vi "AutoExtracOpt.vi"() -> ()   [LabVIEW 2020]
uses:
  <vilib>/NI/Modbus Library/API/Master/Modbus Master.lvclass
  <vilib>/userdefined/High Color/IMAQdx.ctl
  subvi/status/StopSoftware.vi
  subvi/status/Tip_No_1000.vi
  subvi/status/Vial_No.vi
  subvi/status/Tip_No_300.vi
  subvi/status/Liquid_List.vi
  subvi/status/Log.vi
  subvi/status/LogCSVName.vi
  subvi/status/ExtracOptOperations.vi
  subvi/status/ExtracOptDeviceStatus.vi
  subvi/status/ExtracOptTaskStatus.vi
  subvi/status/ExtracOptTaskId.vi
  subvi/status/ExtracOptConversationId.vi
  subvi/status/EmergencyStop.vi
  subvi/status/ExtracOptCommand.vi
  subvi/HitBot/Robot-HL/small_scara_interface/small_scara_interface.lvlib
panel:
  out "ExtracOptDeviceStatus":string
  out "ExtracOptOperations":string
  out "ExtracOptConversationId":string
  out "ExtracOptTaskId":string
  out "Current_1000 uL_Tip_No":i32
  out "Current_300 uL_Tip_No":i32
  out "Current_Vial_No":i32
  out "Current_Log":string
  in  "Device_Log":i32(listbox)
  in  "StopSoftware":bool
  out "DK-CoverSwitcher_TCP":refnum<k5>
  out "DK-Gripper_TCP":refnum<class "Modbus Master.lvclass">
  in  "Control":enum32{"Auto", "Manual", "System", "Photo"}(tab)
  in  "9. End_Extraction 2":bool
  in  "9. End_Extraction":bool
  in  "8. Photo":bool
  in  "7. Shaker":bool
  in  "6. CoverSwitch_To_Extraction_Shaker":bool
  in  "5. CloseCover":bool
  in  "4. CoverSwitch_To_Vial_Storage":bool
  in  "3. OpenCover":bool
  in  "2. Vial_Storage_To_CoverSwitch":bool
  in  "1. DK-CoverSwitcher_Initial":bool
  in  "ExtracOptCommand 2":string="{\"organic_extractants\": [[\"A1\", 1.0], [\"A2\", 2.0]], \"aqueous_extractant\": [\"A3\", 1.0], \"additive\": [\"A4\", 0.0]}"
  in  "Tab Control":enum32{"HitBot76", "DK"}(tab)
  in  "HitBot76_ReadStatus":bool
  in  "HitBot76_Control":bool
  in  "HitBot76_Para":T1
  out "HitBot76_Status":T2
  in  "DK-Gripper_Control":bool
  in  "DK-Gripper_Para":cluster{"mode":string, "distance":i16}
  in  "DK-CoverSwitcher_Control":bool
  in  "DK-CoverSwitcher_Para":cluster{"mode":string}
  in  "PhotoCam":T3="cam1"
  in  "Change_Vial&Tip_No":bool
  in  "Vial_No":i32
  in  "Tip_No_1000":i32
  in  "Tip_No_300":i32
  out "Array":string[][](array[string])
  out "ExtracOptCommand":string
  in  "EmergencyStop":bool
  # "1-10"
  # "开盖模块初始化"
  # "将瓶子抓取到开盖模块，注意瓶子的当前编号"
  # "开瓶盖"
  # "将瓶子从开盖模块抓取回原处，注意瓶子的当前编号"
  # "关瓶盖"
  # "将瓶子从开盖模块抓取到萃取振荡平台"
  # "振荡"
  # "拍照"
  # "结束萃取"
  # "结束萃取"
  # "→ Y"
  # "mode = 0 正常运行\nmode = 1 切换坐标系\nmode = 2 控制夹爪 x\n表示行程0-20"
  # "89"
  # "1"
  # "4"
  # "2"
  # "→"
  # "→"
  # "1"
  # "3"
  # "8"
  # "96"
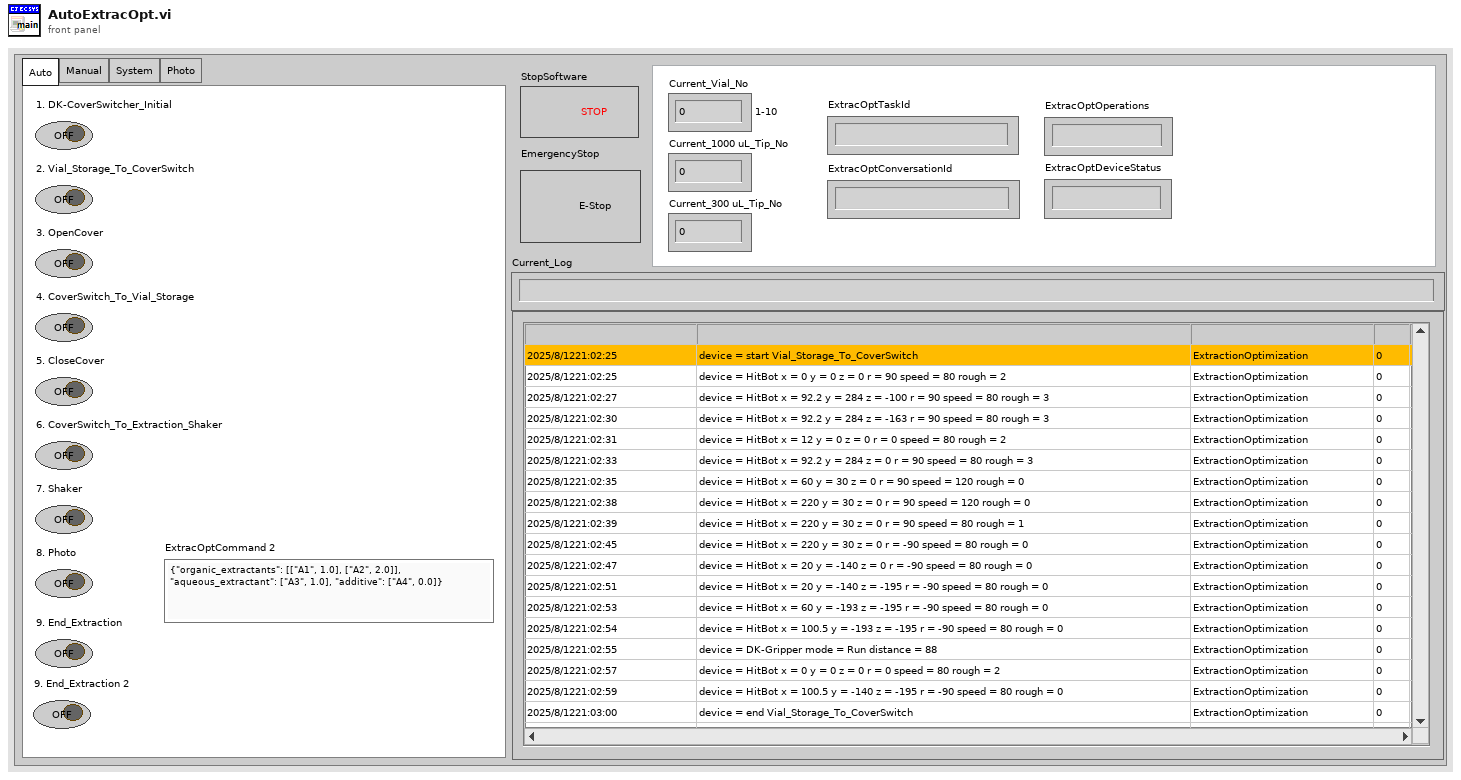
[diagram p1: front panel]
types:
  T1 = cluster{"x":dbl, "y":dbl, "z":dbl, "r":dbl, "speed":dbl, "mode":i32}
  T2 = cluster{"x":sgl, "y":sgl, "z":sgl, "angle1":sgl, "angle2":sgl, "rotation":sgl}
  T3 = typedef "IMAQdx.ctl" = refnum<k21>
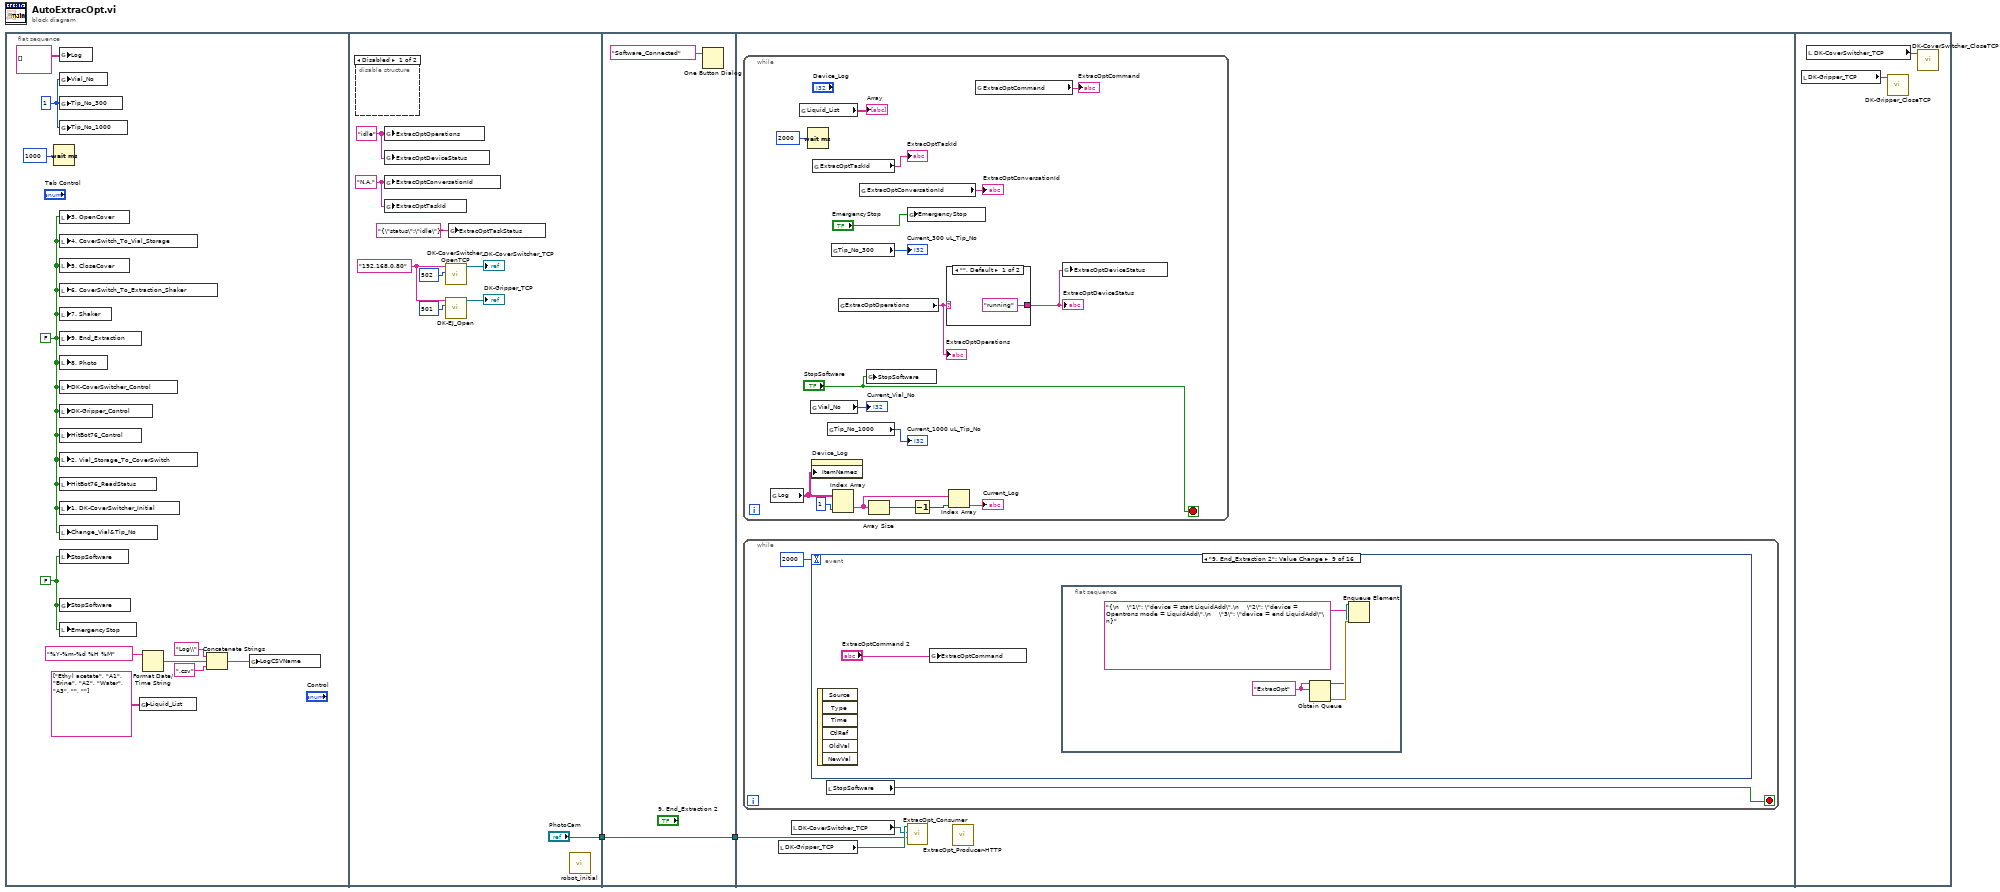
[diagram p0: block diagram]
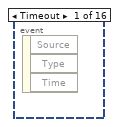
[diagram p3: hidden frame]
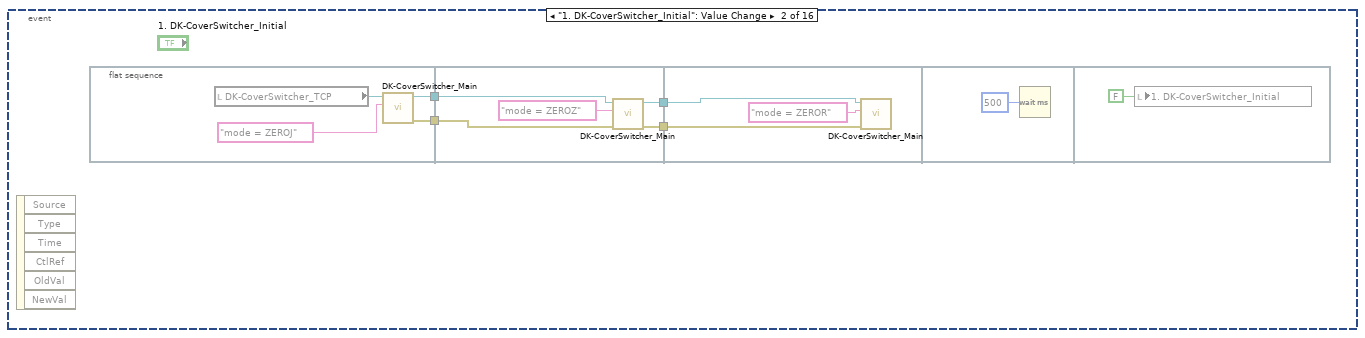
[diagram p4: hidden frame]
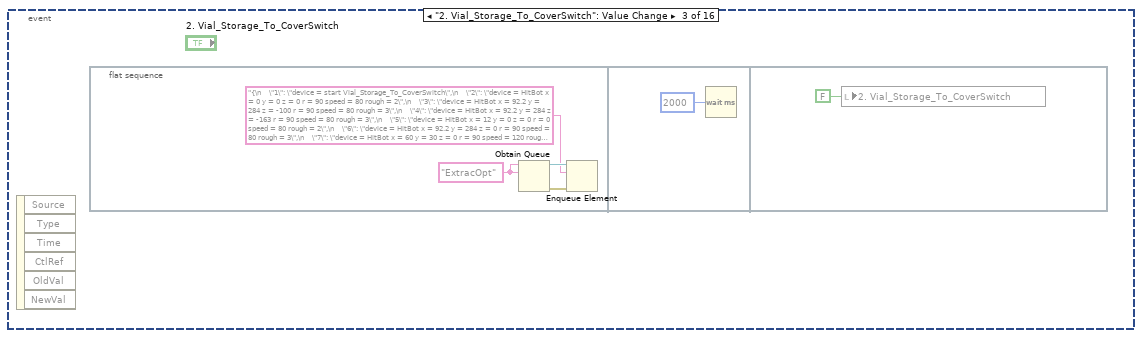
[diagram p5: hidden frame]
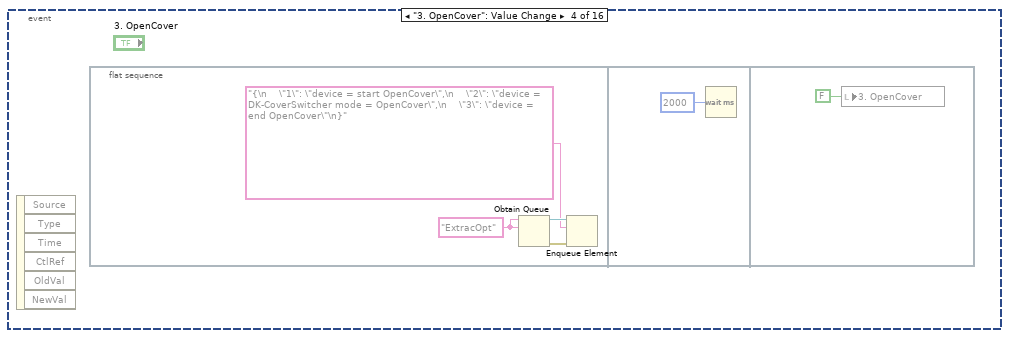
[diagram p6: hidden frame]
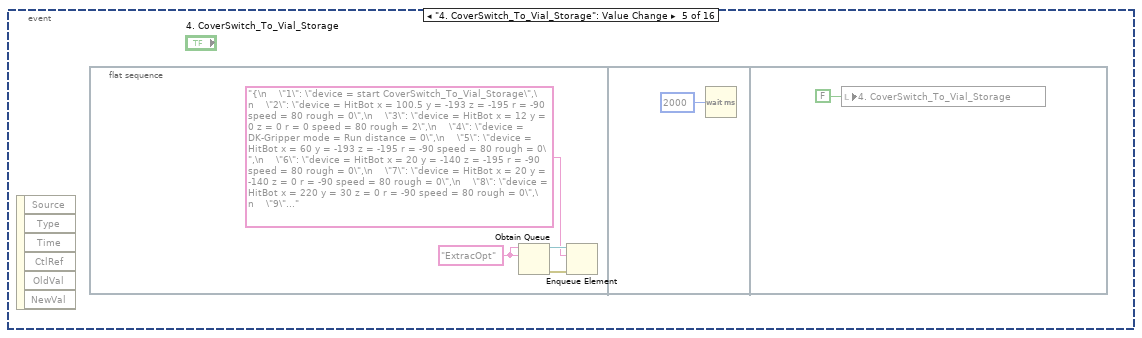
[diagram p7: hidden frame]
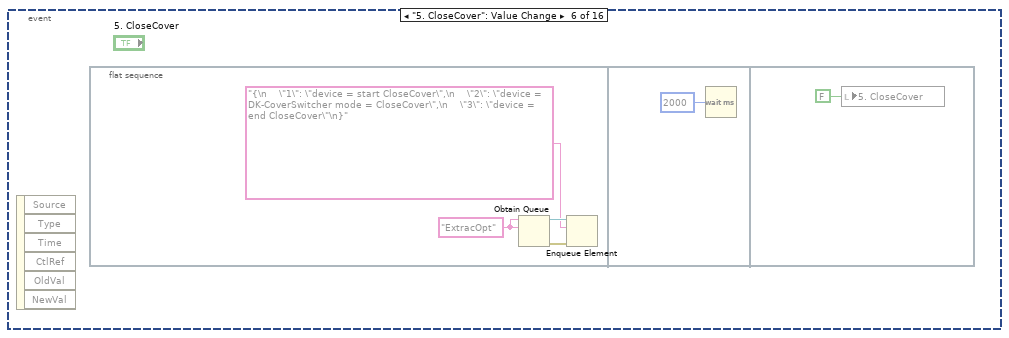
[diagram p8: hidden frame]
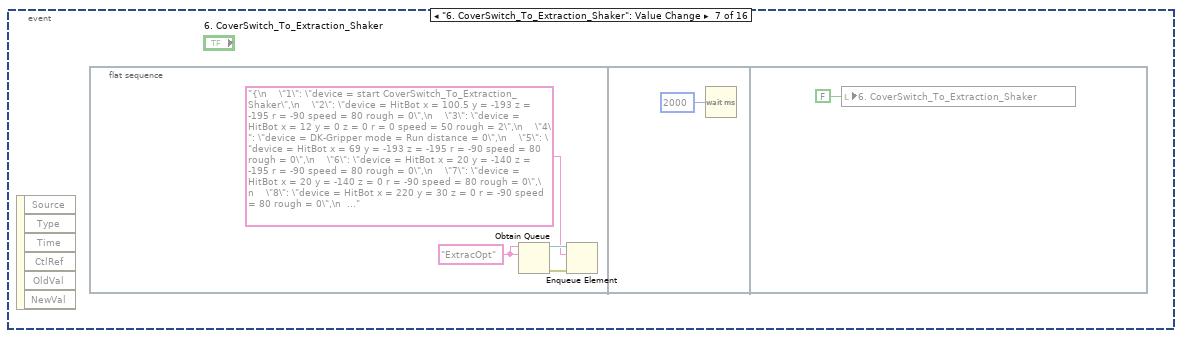
[diagram p9: hidden frame]
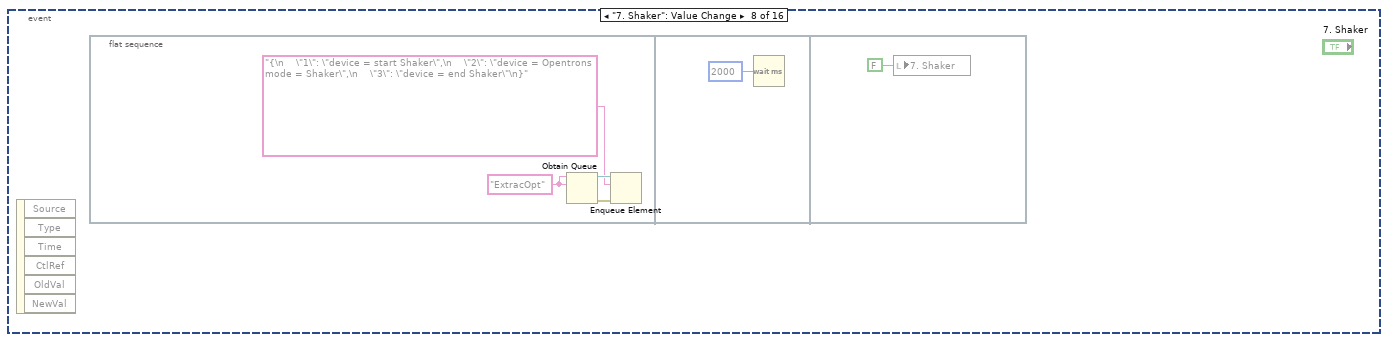
[diagram p10: hidden frame]
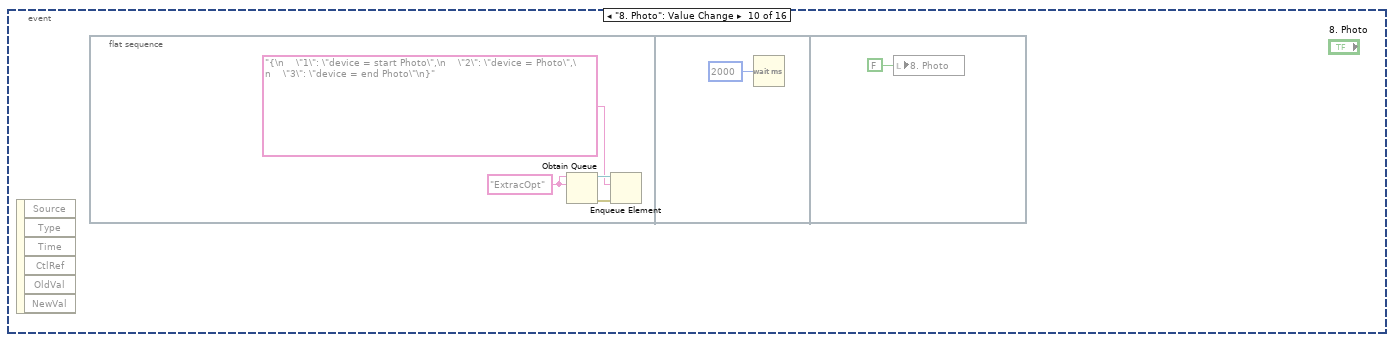
[diagram p11: hidden frame]
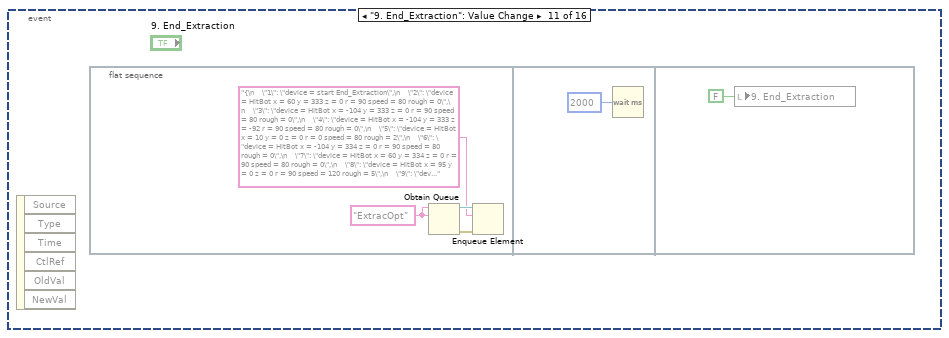
[diagram p12: hidden frame]
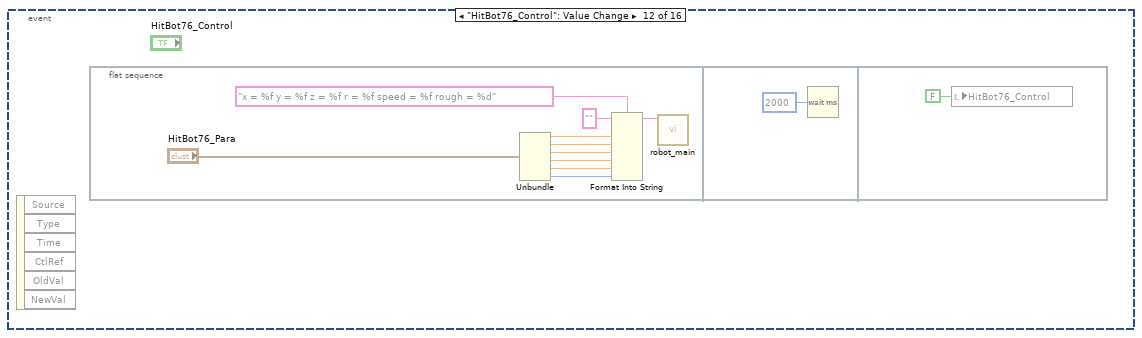
[diagram p13: hidden frame]
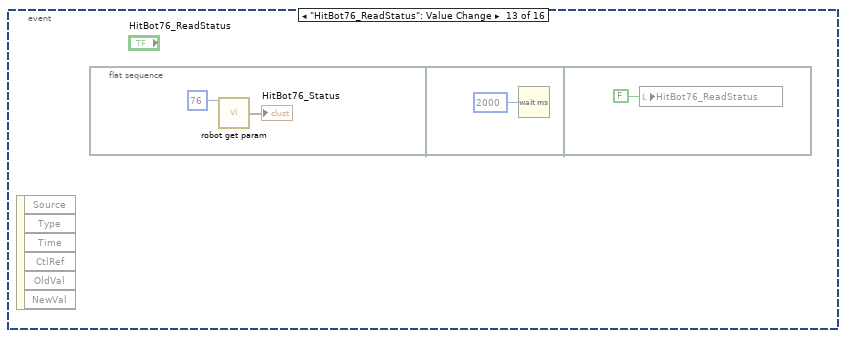
[diagram p14: hidden frame]
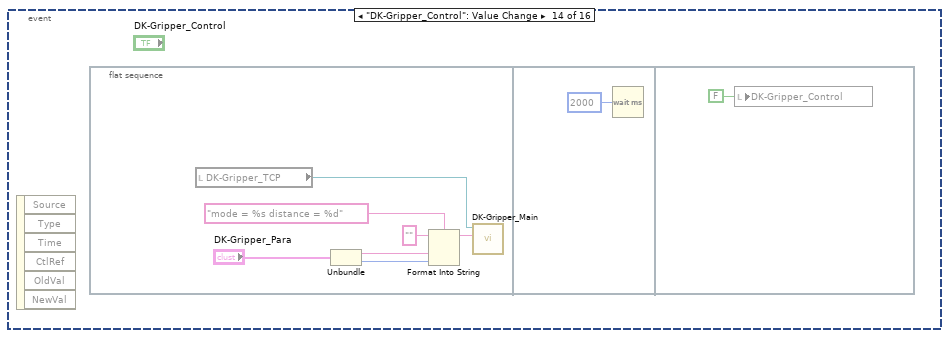
[diagram p15: hidden frame]
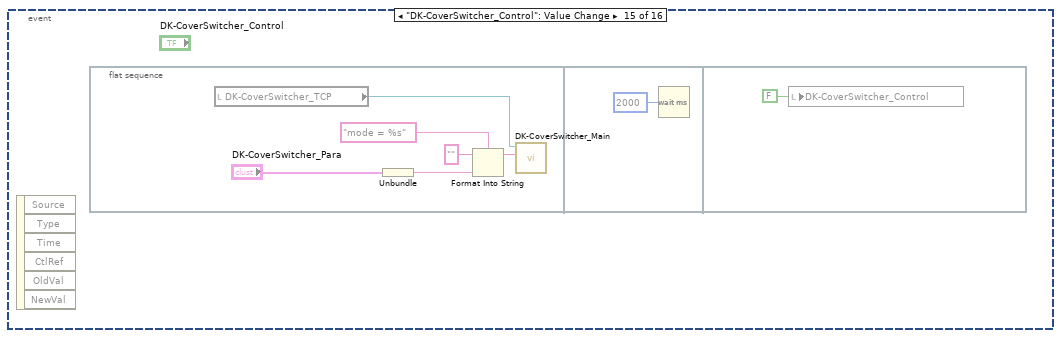
[diagram p16: hidden frame]
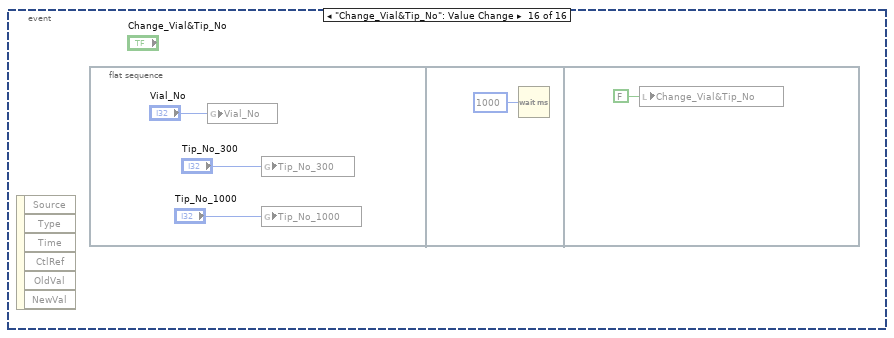
[diagram p17: hidden frame]
diagram:
  n1 = flat-sequence {
    tunnel: ["PhotoCam"] -> w2
    tunnel: w2 -> [w23]
    tunnel: [w23] -> w1
    tunnel: w1 -> [w25]
    frame #0 {
      w3 = FALSE ("Boolean")
      w11 = 1 ("Vial_No")
      w4 = FALSE ("stop software")
      n2 = Wait (ms)(milliseconds to wait=u32 1000) -> ()  [unwired: 1 out]
      n3 = global write "Log.vi" "Log"(string[][] [] ("Log")) -> ()
      n4 = global write "Vial_No.vi" "Vial_No"(w11) -> ()
      n5 = global write "Tip_No_300.vi" "Tip_No_300"(w11) -> ()
      n6 = global write "Tip_No_1000.vi" "Tip_No_1000"(w11) -> ()
      n7 = local write "3. OpenCover"(w3) -> ()
      n8 = local write "4. CoverSwitch_To_Vial_Storage"(w3) -> ()
      n9 = local write "5. CloseCover"(w3) -> ()
      n10 = local write "6. CoverSwitch_To_Extraction_Shaker"(w3) -> ()
      n11 = local write "7. Shaker"(w3) -> ()
      n12 = local write "9. End_Extraction"(w3) -> ()
      n13 = local write "8. Photo"(w3) -> ()
      n14 = local write "DK-CoverSwitcher_Control"(w3) -> ()
      n15 = local write "DK-Gripper_Control"(w3) -> ()
      n16 = local write "HitBot76_Control"(w3) -> ()
      n17 = local write "2. Vial_Storage_To_CoverSwitch"(w3) -> ()
      n18 = local write "HitBot76_ReadStatus"(w3) -> ()
      n19 = local write "1. DK-CoverSwitcher_Initial"(w3) -> ()
      n20 = local write "Change_Vial&Tip_No"(w3) -> ()
      n21 = local write "StopSoftware"(w4) -> ()
      n22 = global write "StopSoftware.vi" "StopSoftware"(w4) -> ()
      n23 = local write "EmergencyStop"(w4) -> ()
      n24 = global write "Liquid_List.vi" "Liquid_List"(string[][] [["Ethyl acetate", "A1"], ["Brine", "A2"], ["Water", "A3"], ["", ""]] ("Liquid_List")) -> ()
      n25 = Format Date/Time String(time format string (%c)="%Y-%m-%d %H %M") -> (date/time string=w10:string)  [unwired: 2 in]
      n26 = Concatenate Strings("Log\\" ("string"), w10, ".csv" ("string")) -> (w9:string)
      n27 = global write "LogCSVName.vi" "LogCSVName"(w9) -> ()
    }
    frame #1 {
      w14 = "N.A." ("ReactorTemp")
      w16 = "idle" ("Operations")
      w21 = "192.168.0.80" ("address")
      n28 = disable-structure shown="Disabled" {
        frame Disabled {
        }
        frame Enabled {
        }
      }
      n29 = global write "ExtracOptOperations.vi" "ExtracOptOperations"(w16) -> ()
      n30 = global write "ExtracOptDeviceStatus.vi" "ExtracOptDeviceStatus"(w16) -> ()
      n31 = global write "ExtracOptConversationId.vi" "ExtracOptConversationId"(w14) -> ()
      n32 = global write "ExtracOptTaskId.vi" "ExtracOptTaskId"(w14) -> ()
      n33 = call "DK-CoverSwitcher_OpenTCP.vi"("remote port"=u16 502, "address"=w21) -> ("connection ID"=→"DK-CoverSwitcher_TCP":refnum<k5>)  [unwired: 8 in, 1 out]
      n34 = call "DK-EJ_Open.vi"("port (502)"=u16 501, "address"=w21) -> ("Modbus master out"=→"DK-Gripper_TCP":refnum<class "Modbus Master.lvclass">)  [unwired: 8 in, 1 out]
      n35 = global write "ExtracOptTaskStatus.vi" "ExtracOptTaskStatus"("{\"status\":\"idle\"}" ("ReactionImagePath")) -> ()
      n36 = call "robot_initial.vi"() -> ()  [unwired: 12 in]
    }
    frame #2 {
      n37 = One Button Dialog(message="Software_Connected") -> ()  [unwired: 1 in, 1 out]
    }
    frame #3 {
      n38 = while {
        stop <- "StopSoftware" stop-if-true
        n39 = global read "Log.vi" "Log"() -> (w145:string[][])
        n40 = global read "Liquid_List.vi" "Liquid_List"() -> (→"Array":string[][])
        n41 = Wait (ms)(milliseconds to wait=u32 2000) -> ()  [unwired: 1 out]
        n42 = global read "Vial_No.vi" "Vial_No"() -> (→"Current_Vial_No":i32)
        n43 = property on="Device_Log" class="MCListbox (strict)"("ItemNames"=w145) -> ()  [unwired: 2 in, 2 out]
        n44 = global read "ExtracOptTaskId.vi" "ExtracOptTaskId"() -> (→"ExtracOptTaskId":string)
        n45 = global read "Tip_No_1000.vi" "Tip_No_1000"() -> (→"Current_1000 uL_Tip_No":i32)
        n46 = global read "Tip_No_300.vi" "Tip_No_300"() -> (→"Current_300 uL_Tip_No":i32)
        n47 = Index Array(array=w145, index (col)=1 ("index (row)")) -> (element=w150:string[])  [unwired: 1 in]
        n48 = global read "ExtracOptOperations.vi" "ExtracOptOperations"() -> (w141:string)
        "ExtracOptOperations" <- w141
        n49 = global read "ExtracOptConversationId.vi" "ExtracOptConversationId"() -> (→"ExtracOptConversationId":string)
        n50 = global write "StopSoftware.vi" "StopSoftware"("StopSoftware") -> ()
        n51 = Array Size(array=w150) -> (size(s)=w147:i32)
        n52 = global write "EmergencyStop.vi" "EmergencyStop"("EmergencyStop") -> ()
        n53 = Decrement(x=w147) -> (x-1=w146:i32)
        n54 = case shown="\"\", Default" w141 {
          selector: w141 -> [_ w158]
          tunnel: ["running" ("ReactionDeviceStatus") w158] -> w140
          frame "", Default {
          }
          frame "idle" {
          }
        }
        "ExtracOptDeviceStatus" <- w140
        n55 = Index Array(array=w150, index=w146) -> (element=→"Current_Log":string)
        n56 = global read "ExtracOptCommand.vi" "ExtracOptCommand"() -> (→"ExtracOptCommand":string)
        n57 = global write "ExtracOptDeviceStatus.vi" "ExtracOptDeviceStatus"(w140) -> ()
      }
      n58 = while {
        stop <- w29 stop-if-true
        n59 = event shown="[8] \"9. End_Extraction 2\": Value Change" {
          selector: _ -> [_ _ _ _ _ _ _ _ _ _ _ _ _ _ _ _]
          dyn-events: _ -> [_ _ _ _ _ _ _ _ _ _ _ _ _ _ _ _]
          timeout: 2000 -> [_ _ _ _ _ _ _ _ _ _ _ _ _ _ _ _]
          event Timeout {
            n60 = event-data() -> ()  [unwired: 1 in, 3 out]
          }
          event "1. DK-CoverSwitcher_Initial": Value Change {
            n61 = event-data() -> ()  [unwired: 1 in, 6 out]
            n62 = flat-sequence {
              tunnel: [w35] -> w33
              tunnel: [w34] -> w31
              tunnel: w33 -> [w41]
              tunnel: [w40] -> w32
              tunnel: w31 -> [w39]
              tunnel: [w38] -> w30
              tunnel: w32 -> [w44]
              tunnel: w30 -> [w43]
              frame #0 {
                n63 = local read "DK-CoverSwitcher_TCP"() -> (w36:refnum<k5>)
                n64 = call "DK-CoverSwitcher_Main.vi"("input string"="mode = ZEROJ" ("format string"), "connection ID"=w36) -> ("error out"=w35:errorcluster, "connection ID out"=w34:refnum<k5>)  [unwired: 8 in]
              }
              frame #1 {
                n65 = call "DK-CoverSwitcher_Main.vi"("error in (no error)"=w41, "input string"="mode = ZEROZ" ("format string"), "connection ID"=w39) -> ("error out"=w40:errorcluster, "connection ID out"=w38:refnum<k5>)  [unwired: 7 in]
              }
              frame #2 {
                n66 = call "DK-CoverSwitcher_Main.vi"("error in (no error)"=w44, "input string"="mode = ZEROR" ("format string"), "connection ID"=w43) -> ()  [unwired: 7 in, 2 out]
              }
              frame #3 {
                n67 = Wait (ms)(milliseconds to wait=u32 500) -> ()  [unwired: 1 out]
              }
              frame #4 {
                n68 = local write "1. DK-CoverSwitcher_Initial"(FALSE ("1. DK-CoverSwitcher_Initial")) -> ()
              }
            }
          }
          event "2. Vial_Storage_To_CoverSwitch": Value Change {
            n69 = event-data() -> ()  [unwired: 1 in, 6 out]
            n70 = flat-sequence {
              frame #0 {
                w48 = "ExtracOpt" ("name (unnamed)")
                n71 = Obtain Queue(name (unnamed)=w48, element data type=w48) -> (queue out=w50:refnum<queue>, error out=w51:errorcluster)  [unwired: 3 in, 1 out]
                n72 = Enqueue Element(queue=w50, element="{\n    \"1\": \"device = start Vial_Storage_To_CoverSwitch\",\n    \"2\": \"device = HitBot x = 0 y = 0 z = 0 r = 90 speed = 80 rough = 2\",\n    \"3\": \"device = HitBot x = 92.2 y = 284 z = -100 r = 90 speed = 80 rough = 3\",\n    \"4\": \"device = HitBot x = 92.2 y = 284 z = -163 r = 90 speed = 80 rough = 3\",\n    \"5\": \"device = HitBot x = 12 y = 0 z = 0 r = 0 speed = 80 rough = 2\",\n    \"6\": \"device = HitBot x = 92.2 y = 284 z = 0 r = 90 speed = 80 rough = 3\",\n    \"7\": \"device = HitBot x = 60 y = 30 z = 0 r = 90 speed = 120 rough = 0\",\n    \"8\": \"device = HitBot x = 220 y = 30 z = 0 r = 90 speed = 120 rough = 0\",\n    \"9\": \"device = HitBot x = 220 y = 30 z = 0 r = 90 speed = 80 rough = 1\",\n    \"10\": \"device = HitBot x = 220 y = 30 z = 0 r = -90 speed = 80 rough = 0\",\n    \"11\": \"device = HitBot x = 20 y = -140 z = 0 r = -90 speed = 80 rough = 0\",\n    \"12\": \"device = HitBot x = 20 y = -140 z = -195 r = -90 speed = 80 rough = 0\",\n    \"13\": \"device = HitBot x = 60 y = -193 z = -195 r = -90 speed = 80 rough = 0\",\n    \"14\": \"device = HitBot x = 100.5 y = -193 z = -195 r = -90 speed = 80 rough = 0\",\n    \"15\": \"device = DK-Gripper mode = Run distance = 88\",\n    \"16\": \"device = HitBot x = 0 y = 0 z = 0 r = 0 speed = 80 rough = 2\",\n    \"17\": \"device = HitBot x = 100.5 y = -140 z = -195 r = -90 speed = 80 rough = 0\",\n    \"18\": \"device = end Vial_Storage_To_CoverSwitch\"\n}" ("JSON string"), error in (no error)=w51) -> ()  [unwired: 1 in, 3 out]
              }
              frame #1 {
                n73 = Wait (ms)(milliseconds to wait=u32 2000) -> ()  [unwired: 1 out]
              }
              frame #2 {
                n74 = local write "2. Vial_Storage_To_CoverSwitch"(FALSE ("2. Vial_Storage_To_CoverSwitch")) -> ()
              }
            }
          }
          event "3. OpenCover": Value Change {
            n75 = event-data() -> ()  [unwired: 1 in, 6 out]
            n76 = flat-sequence {
              frame #0 {
                w54 = "ExtracOpt" ("name (unnamed)")
                n77 = Obtain Queue(name (unnamed)=w54, element data type=w54) -> (queue out=w56:refnum<queue>, error out=w57:errorcluster)  [unwired: 3 in, 1 out]
                n78 = Enqueue Element(queue=w56, element="{\n    \"1\": \"device = start OpenCover\",\n    \"2\": \"device = DK-CoverSwitcher mode = OpenCover\",\n    \"3\": \"device = end OpenCover\"\n}" ("JSON string"), error in (no error)=w57) -> ()  [unwired: 1 in, 3 out]
              }
              frame #1 {
                n79 = Wait (ms)(milliseconds to wait=u32 2000) -> ()  [unwired: 1 out]
              }
              frame #2 {
                n80 = local write "3. OpenCover"(FALSE ("3. OpenCover")) -> ()
              }
            }
          }
          event "4. CoverSwitch_To_Vial_Storage": Value Change {
            n81 = event-data() -> ()  [unwired: 1 in, 6 out]
            n82 = flat-sequence {
              frame #0 {
                w60 = "ExtracOpt" ("name (unnamed)")
                n83 = Obtain Queue(name (unnamed)=w60, element data type=w60) -> (queue out=w62:refnum<queue>, error out=w63:errorcluster)  [unwired: 3 in, 1 out]
                n84 = Enqueue Element(queue=w62, element="{\n    \"1\": \"device = start CoverSwitch_To_Vial_Storage\",\n    \"2\": \"device = HitBot x = 100.5 y = -193 z = -195 r = -90 speed = 80 rough = 0\",\n    \"3\": \"device = HitBot x = 12 y = 0 z = 0 r = 0 speed = 80 rough = 2\",\n    \"4\": \"device = DK-Gripper mode = Run distance = 0\",\n    \"5\": \"device = HitBot x = 60 y = -193 z = -195 r = -90 speed = 80 rough = 0\",\n    \"6\": \"device = HitBot x = 20 y = -140 z = -195 r = -90 speed = 80 rough = 0\",\n    \"7\": \"device = HitBot x = 20 y = -140 z = 0 r = -90 speed = 80 rough = 0\",\n    \"8\": \"device = HitBot x = 220 y = 30 z = 0 r = -90 speed = 80 rough = 0\",\n    \"9\": \"device = HitBot x = 220 y = 30 z = 0 r = 90 speed = 80 rough = 0\",\n    \"10\": \"device = HitBot x = 220 y = 30 z = 0 r = 90 speed = 80 rough = 1\",\n    \"11\": \"device = HitBot x = 60 y = 30 z = 0 r = 90 speed = 120 rough = 0\",\n    \"12\": \"device = HitBot x = 92.2 y = 284 z = 0 r = 90 speed = 80 rough = 3\",\n    \"13\": \"device = HitBot x = 92.2 y = 284 z = -163 r = 90 speed = 80 rough = 3\",\n    \"14\": \"device = HitBot x = 0 y = 0 z = 0 r = 0 speed = 80 rough = 2\",\n    \"15\": \"device = HitBot x = 92.2 y = 284 z = -100 r = 90 speed = 120 rough = 3\",\n    \"16\": \"device = HitBot x = 60 y = 100 z = 0 r = 90 speed = 120 rough = 0\",\n    \"17\": \"device = end CoverSwitch_To_Vial_Storage\"\n}" ("JSON string"), error in (no error)=w63) -> ()  [unwired: 1 in, 3 out]
              }
              frame #1 {
                n85 = Wait (ms)(milliseconds to wait=u32 2000) -> ()  [unwired: 1 out]
              }
              frame #2 {
                n86 = local write "4. CoverSwitch_To_Vial_Storage"(FALSE ("4. CoverSwitch_To_Vial_Storage")) -> ()
              }
            }
          }
          event "5. CloseCover": Value Change {
            n87 = event-data() -> ()  [unwired: 1 in, 6 out]
            n88 = flat-sequence {
              frame #0 {
                w66 = "ExtracOpt" ("name (unnamed)")
                n89 = Obtain Queue(name (unnamed)=w66, element data type=w66) -> (queue out=w68:refnum<queue>, error out=w69:errorcluster)  [unwired: 3 in, 1 out]
                n90 = Enqueue Element(queue=w68, element="{\n    \"1\": \"device = start CloseCover\",\n    \"2\": \"device = DK-CoverSwitcher mode = CloseCover\",\n    \"3\": \"device = end CloseCover\"\n}" ("JSON string"), error in (no error)=w69) -> ()  [unwired: 1 in, 3 out]
              }
              frame #1 {
                n91 = Wait (ms)(milliseconds to wait=u32 2000) -> ()  [unwired: 1 out]
              }
              frame #2 {
                n92 = local write "5. CloseCover"(FALSE ("5. CloseCover")) -> ()
              }
            }
          }
          event "6. CoverSwitch_To_Extraction_Shaker": Value Change {
            n93 = event-data() -> ()  [unwired: 1 in, 6 out]
            n94 = flat-sequence {
              frame #0 {
                w72 = "ExtracOpt" ("name (unnamed)")
                n95 = Obtain Queue(name (unnamed)=w72, element data type=w72) -> (queue out=w74:refnum<queue>, error out=w75:errorcluster)  [unwired: 3 in, 1 out]
                n96 = Enqueue Element(queue=w74, element="{\n    \"1\": \"device = start CoverSwitch_To_Extraction_Shaker\",\n    \"2\": \"device = HitBot x = 100.5 y = -193 z = -195 r = -90 speed = 80 rough = 0\",\n    \"3\": \"device = HitBot x = 12 y = 0 z = 0 r = 0 speed = 50 rough = 2\",\n    \"4\": \"device = DK-Gripper mode = Run distance = 0\",\n    \"5\": \"device = HitBot x = 69 y = -193 z = -195 r = -90 speed = 80 rough = 0\",\n    \"6\": \"device = HitBot x = 20 y = -140 z = -195 r = -90 speed = 80 rough = 0\",\n    \"7\": \"device = HitBot x = 20 y = -140 z = 0 r = -90 speed = 80 rough = 0\",\n    \"8\": \"device = HitBot x = 220 y = 30 z = 0 r = -90 speed = 80 rough = 0\",\n    \"9\": \"device = HitBot x = 220 y = 30 z = 0 r = 90 speed = 80 rough = 0\",\n    \"10\": \"device = HitBot x = 220 y = 30 z = 0 r = 90 speed = 80 rough = 1\",\n    \"11\": \"device = HitBot x = 60 y = 30 z = 0 r = 90 speed = 120 rough = 0\",\n    \"12\": \"device = HitBot x = 60 y = 333.7 z = 0 r = 90 speed = 80 rough = 0\",\n    \"13\": \"device = HitBot x = -104.5 y = 333.7 z = 0 r = 90 speed = 80 rough = 0\",   \n    \"14\": \"device = HitBot x = -104.5 y = 333.7 z = -88 r = 90 speed = 40 rough = 0\",\n    \"15\": \"device = HitBot x = 0 y = 0 z = 0 r = 0 speed = 80 rough = 2\",\n    \"16\": \"device = HitBot x = -104.5 y = 333.7 z = 0 r = 90 speed = 40 rough = 0\",\n    \"17\": \"device = HitBot x = 60 y = 334 z = 0 r = 90 speed = 80 rough = 0\",\n    \"18\": \"device = HitBot x = 60 y = 100 z = 0 r = 90 speed = 120 rough = 0\",\n    \"19\": \"device = end CoverSwitch_To_Extraction_Shaker\"\n}" ("JSON string"), error in (no error)=w75) -> ()  [unwired: 1 in, 3 out]
              }
              frame #1 {
                n97 = Wait (ms)(milliseconds to wait=u32 2000) -> ()  [unwired: 1 out]
              }
              frame #2 {
                n98 = local write "6. CoverSwitch_To_Extraction_Shaker"(FALSE ("6. CoverSwitch_To_Extraction_Shaker")) -> ()
              }
            }
          }
          event "7. Shaker": Value Change {
            n99 = event-data() -> ()  [unwired: 1 in, 6 out]
            n100 = flat-sequence {
              frame #0 {
                w79 = "ExtracOpt" ("name (unnamed)")
                n101 = Obtain Queue(name (unnamed)=w79, element data type=w79) -> (queue out=w80:refnum<queue>, error out=w81:errorcluster)  [unwired: 3 in, 1 out]
                n102 = Enqueue Element(queue=w80, element="{\n    \"1\": \"device = start Shaker\",\n    \"2\": \"device = Opentrons mode = Shaker\",\n    \"3\": \"device = end Shaker\"\n}" ("JSON string"), error in (no error)=w81) -> ()  [unwired: 1 in, 3 out]
              }
              frame #1 {
                n103 = Wait (ms)(milliseconds to wait=u32 2000) -> ()  [unwired: 1 out]
              }
              frame #2 {
                n104 = local write "7. Shaker"(FALSE ("7. Shaker")) -> ()
              }
            }
          }
          event "9. End_Extraction 2": Value Change {
            n105 = event-data() -> ()  [unwired: 1 in, 6 out]
            n106 = global write "ExtracOptCommand.vi" "ExtracOptCommand"("ExtracOptCommand 2") -> ()
            n107 = flat-sequence {
              frame #0 {
                w87 = "ExtracOpt" ("name (unnamed)")
                n108 = Obtain Queue(name (unnamed)=w87, element data type=w87) -> (queue out=w86:refnum<queue>, error out=w88:errorcluster)  [unwired: 3 in, 1 out]
                n109 = Enqueue Element(queue=w86, element="{\n    \"1\": \"device = start LiquidAdd\",\n    \"2\": \"device = Opentrons mode = LiquidAdd\",\n    \"3\": \"device = end LiquidAdd\"\n}" ("JSON string"), error in (no error)=w88) -> ()  [unwired: 1 in, 3 out]
              }
            }
          }
          event "8. Photo": Value Change {
            n110 = event-data() -> ()  [unwired: 1 in, 6 out]
            n111 = flat-sequence {
              frame #0 {
                w90 = "ExtracOpt" ("name (unnamed)")
                n112 = Obtain Queue(name (unnamed)=w90, element data type=w90) -> (queue out=w91:refnum<queue>, error out=w92:errorcluster)  [unwired: 3 in, 1 out]
                n113 = Enqueue Element(queue=w91, element="{\n    \"1\": \"device = start Photo\",\n    \"2\": \"device = Photo\",\n    \"3\": \"device = end Photo\"\n}" ("JSON string"), error in (no error)=w92) -> ()  [unwired: 1 in, 3 out]
              }
              frame #1 {
                n114 = Wait (ms)(milliseconds to wait=u32 2000) -> ()  [unwired: 1 out]
              }
              frame #2 {
                n115 = local write "8. Photo"(FALSE ("8. Photo")) -> ()
              }
            }
          }
          event "9. End_Extraction": Value Change {
            n116 = event-data() -> ()  [unwired: 1 in, 6 out]
            n117 = flat-sequence {
              frame #0 {
                w96 = "ExtracOpt" ("name (unnamed)")
                n118 = Obtain Queue(name (unnamed)=w96, element data type=w96) -> (queue out=w97:refnum<queue>, error out=w98:errorcluster)  [unwired: 3 in, 1 out]
                n119 = Enqueue Element(queue=w97, element="{\n    \"1\": \"device = start End_Extraction\",\n    \"2\": \"device = HitBot x = 60 y = 333 z = 0 r = 90 speed = 80 rough = 0\",\n    \"3\": \"device = HitBot x = -104 y = 333 z = 0 r = 90 speed = 80 rough = 0\",\n    \"4\": \"device = HitBot x = -104 y = 333 z = -92 r = 90 speed = 80 rough = 0\",\n    \"5\": \"device = HitBot x = 10 y = 0 z = 0 r = 0 speed = 80 rough = 2\",\n    \"6\": \"device = HitBot x = -104 y = 334 z = 0 r = 90 speed = 80 rough = 0\",\n    \"7\": \"device = HitBot x = 60 y = 334 z = 0 r = 90 speed = 80 rough = 0\",\n    \"8\": \"device = HitBot x = 95 y = 0 z = 0 r = 90 speed = 120 rough = 5\",\n    \"9\": \"device = HitBot x = 95 y = 0 z = -232 r = 90 speed = 120 rough = 5\",\n    \"10\": \"device = HitBot x = 0 y = 0 z = 0 r = 0 speed = 80 rough = 2\",\n    \"11\": \"device = HitBot x = 60 y = 100 z = 0 r = 90 speed = 120 rough = 4\",\n    \"12\": \"device = end End_Extraction\"\n}" ("JSON string"), error in (no error)=w98) -> ()  [unwired: 1 in, 3 out]
              }
              frame #1 {
                n120 = Wait (ms)(milliseconds to wait=u32 2000) -> ()  [unwired: 1 out]
              }
              frame #2 {
                n121 = local write "9. End_Extraction"(FALSE ("9. End_Extraction")) -> ()
              }
            }
          }
          event "HitBot76_Control": Value Change {
            n122 = event-data() -> ()  [unwired: 1 in, 6 out]
            n123 = flat-sequence {
              frame #0 {
                n124 = Unbundle("HitBot76_Para") -> ("x"=w107:dbl, "y"=w106:dbl, "z"=w105:dbl, "r"=w104:dbl, "speed"=w103:dbl, "mode"=w102:i32)
                n125 = Format Into String(format string="x = %f y = %f z = %f r = %f speed = %f rough = %d", initial string="", w107, w106, w105, w104, w103, w102) -> (resulting string=w101:string)  [unwired: 1 in, 1 out]
                n126 = call "robot_main.vi"("input string"=w101) -> ()  [unwired: 10 in, 1 out]
              }
              frame #1 {
                n127 = Wait (ms)(milliseconds to wait=u32 2000) -> ()  [unwired: 1 out]
              }
              frame #2 {
                n128 = local write "HitBot76_Control"(FALSE ("HitBot76_Control")) -> ()
              }
            }
          }
          event "HitBot76_ReadStatus": Value Change {
            n129 = event-data() -> ()  [unwired: 1 in, 6 out]
            n130 = flat-sequence {
              frame #0 {
                n131 = call "robot get param.vi"("robot_id"=76) -> ("输出参数簇"=→"HitBot76_Status":T2)  [unwired: 11 in, 3 out]
              }
              frame #1 {
                n132 = Wait (ms)(milliseconds to wait=u32 2000) -> ()  [unwired: 1 out]
              }
              frame #2 {
                n133 = local write "HitBot76_ReadStatus"(FALSE ("HitBot76_QueryStatus")) -> ()
              }
            }
          }
          event "DK-Gripper_Control": Value Change {
            n134 = event-data() -> ()  [unwired: 1 in, 6 out]
            n135 = flat-sequence {
              frame #0 {
                n136 = local read "DK-Gripper_TCP"() -> (w123:refnum<class "Modbus Master.lvclass">)
                n137 = Unbundle("DK-Gripper_Para") -> ("mode"=w118:string, "distance"=w117:i16)
                n138 = Format Into String(format string="mode = %s distance = %d", initial string="", w118, w117) -> (resulting string=w120:string)  [unwired: 1 in, 1 out]
                n139 = call "DK-Gripper_Main.vi"("input string"=w120, "Modbus master in"=w123) -> ()  [unwired: 9 in, 1 out]
              }
              frame #1 {
                n140 = Wait (ms)(milliseconds to wait=u32 2000) -> ()  [unwired: 1 out]
              }
              frame #2 {
                n141 = local write "DK-Gripper_Control"(FALSE ("DK-Gripper_Control")) -> ()
              }
            }
          }
          event "DK-CoverSwitcher_Control": Value Change {
            n142 = event-data() -> ()  [unwired: 1 in, 6 out]
            n143 = flat-sequence {
              frame #0 {
                n144 = local read "DK-CoverSwitcher_TCP"() -> (w126:refnum<k5>)
                n145 = Unbundle("DK-CoverSwitcher_Para") -> ("mode"=w128:string)
                n146 = Format Into String(format string="mode = %s", initial string="", w128) -> (resulting string=w127:string)  [unwired: 1 in, 1 out]
                n147 = call "DK-CoverSwitcher_Main.vi"("input string"=w127, "connection ID"=w126) -> ()  [unwired: 8 in, 2 out]
              }
              frame #1 {
                n148 = Wait (ms)(milliseconds to wait=u32 2000) -> ()  [unwired: 1 out]
              }
              frame #2 {
                n149 = local write "DK-CoverSwitcher_Control"(FALSE ("DK-CoverSwitcher_Control")) -> ()
              }
            }
          }
          event "Change_Vial&Tip_No": Value Change {
            n150 = event-data() -> ()  [unwired: 1 in, 6 out]
            n151 = flat-sequence {
              frame #0 {
                n152 = global write "Vial_No.vi" "Vial_No"("Vial_No") -> ()
                n153 = global write "Tip_No_300.vi" "Tip_No_300"("Tip_No_300") -> ()
                n154 = global write "Tip_No_1000.vi" "Tip_No_1000"("Tip_No_1000") -> ()
              }
              frame #1 {
                n155 = Wait (ms)(milliseconds to wait=u32 1000) -> ()  [unwired: 1 out]
              }
              frame #2 {
                n156 = local write "Change_Vial&Tip_No"(FALSE ("Add_Vial_No")) -> ()
              }
            }
          }
        }
        n157 = local read "StopSoftware"() -> (w29:bool)
      }
      n158 = local read "DK-Gripper_TCP"() -> (w27:refnum<class "Modbus Master.lvclass">)
      n159 = local read "DK-CoverSwitcher_TCP"() -> (w26:refnum<k5>)
      n160 = call "ExtracOpt_Consumer.vi"("front-cam"=w25, "DK-CoverSwitcher-TCP"=w26, "DK-Gripper-TCP"=w27) -> ()  [unwired: 9 in]
      n161 = call "ExtracOpt_Producer-HTTP.vi"() -> ()  [unwired: 12 in]
    }
    frame #4 {
      n162 = local read "DK-Gripper_TCP"() -> (w159:refnum<class "Modbus Master.lvclass">)
      n163 = local read "DK-CoverSwitcher_TCP"() -> (w160:refnum<k5>)
      n164 = call "DK-Gripper_CloseTCP.vi"("Modbus master in"=w159) -> ()  [unwired: 11 in]
      n165 = call "DK-CoverSwitcher_CloseTCP.vi"("connection ID"=w160) -> ()  [unwired: 11 in]
    }
  }
